vi "iTCread.vi"(0 "VISA resource name":refnum<visa-resource-name>, 1 "iTCreadCtrl":T1, 3 "error in (no error)":errorcluster) -> (7 "VISA resource name out":refnum<visa-resource-name>, 8 "number":dbl, 9 "read buffer":string, 10 "error out":errorcluster)   [LabVIEW 2021]
uses:
  controls/iTCreadCtrl.ctl
  <vilib>/regexp/Match Regular Expression.xnode
panel:
  out "read buffer 2":string
  out "after match":string
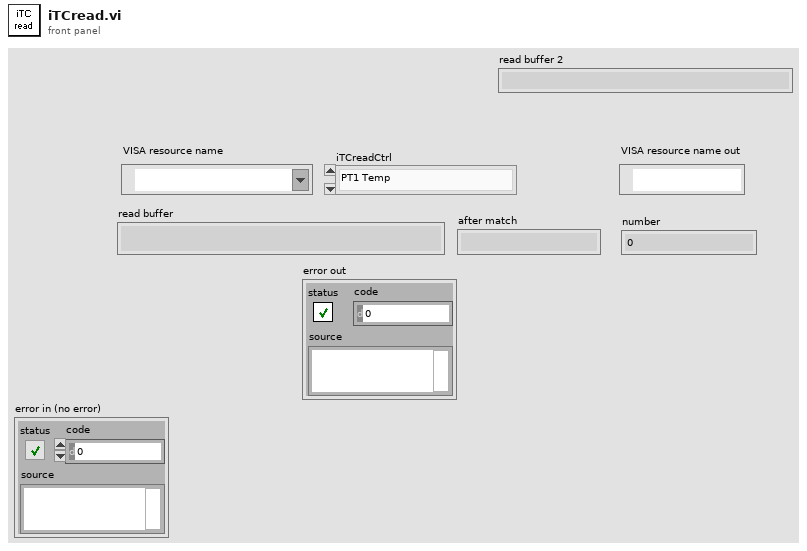
[diagram p1: front panel]
types:
  T1 = typedef "iTCreadCtrl.ctl" = enum16{"PT1 Temp", "PT2 Temp", "Sample Temp", "VTI Temp", "Needle Valve", "VTI Heater Power", "Sample Heater Power", "VTI Pressure"}
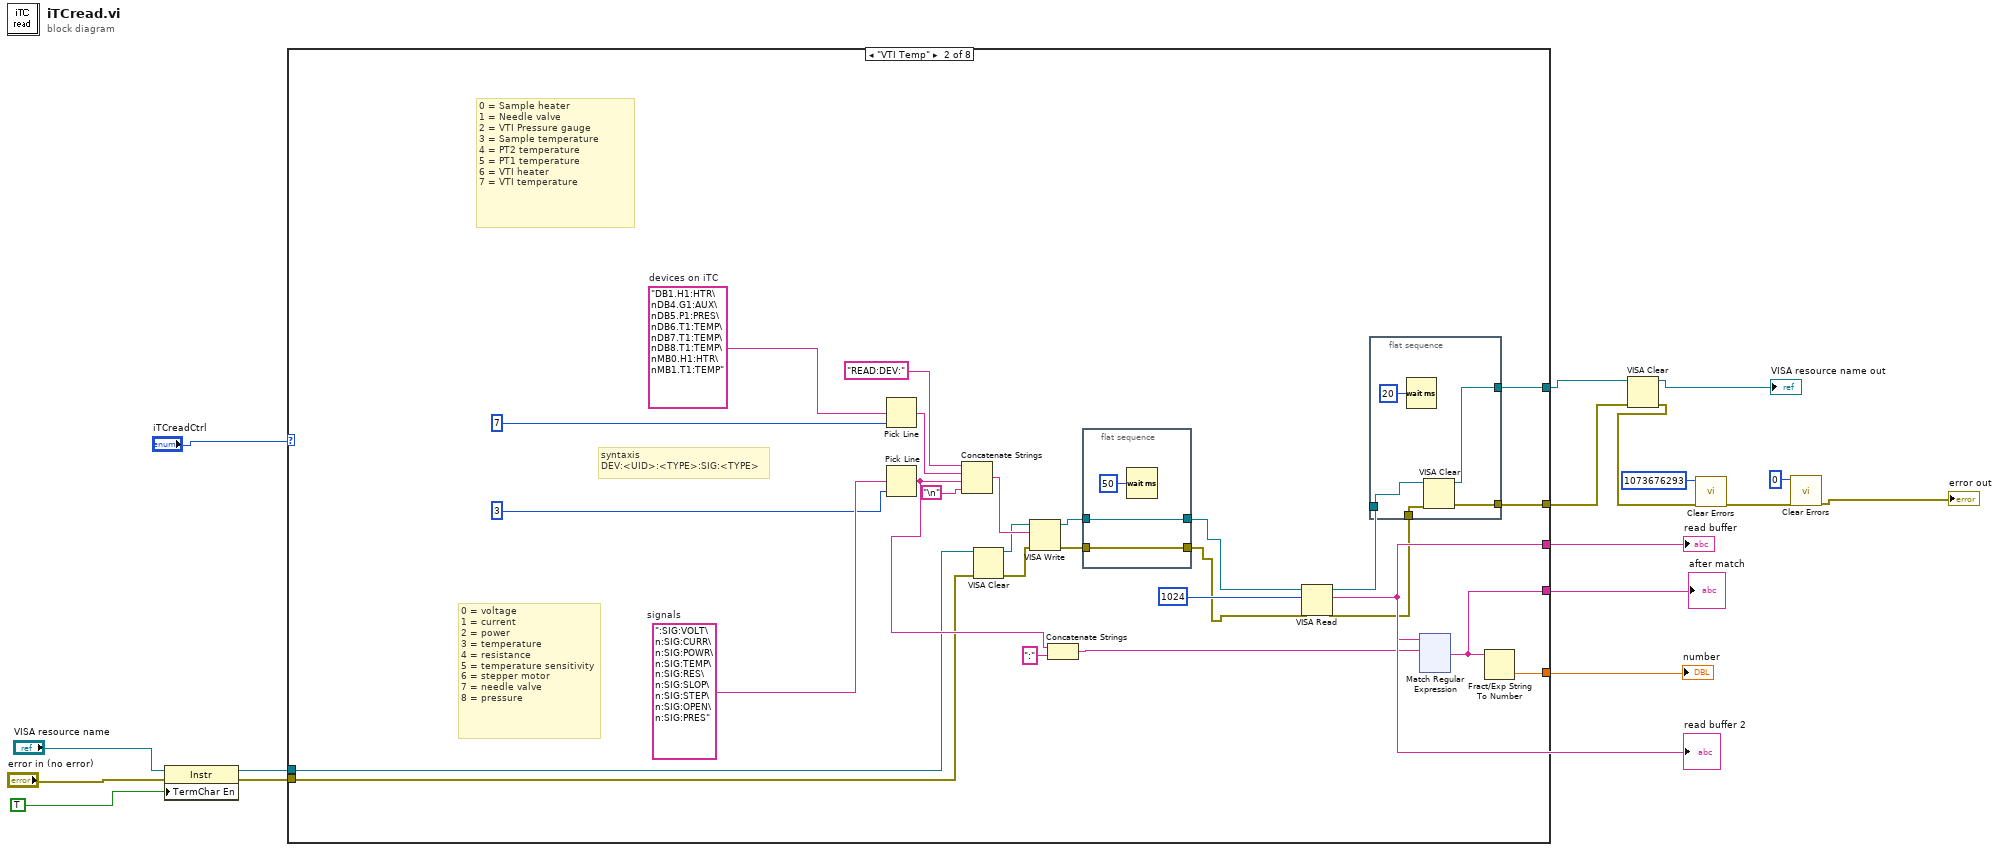
[diagram p0: block diagram]
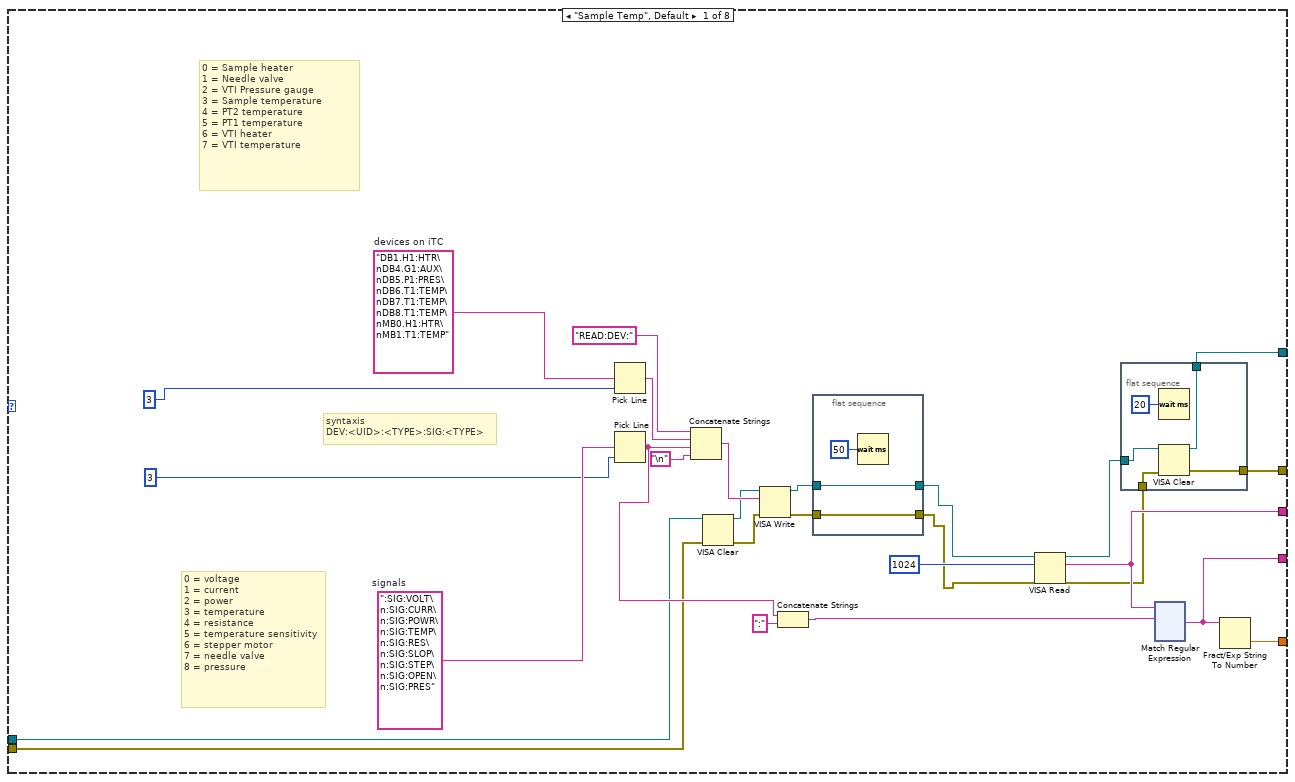
[diagram p2: hidden frame]
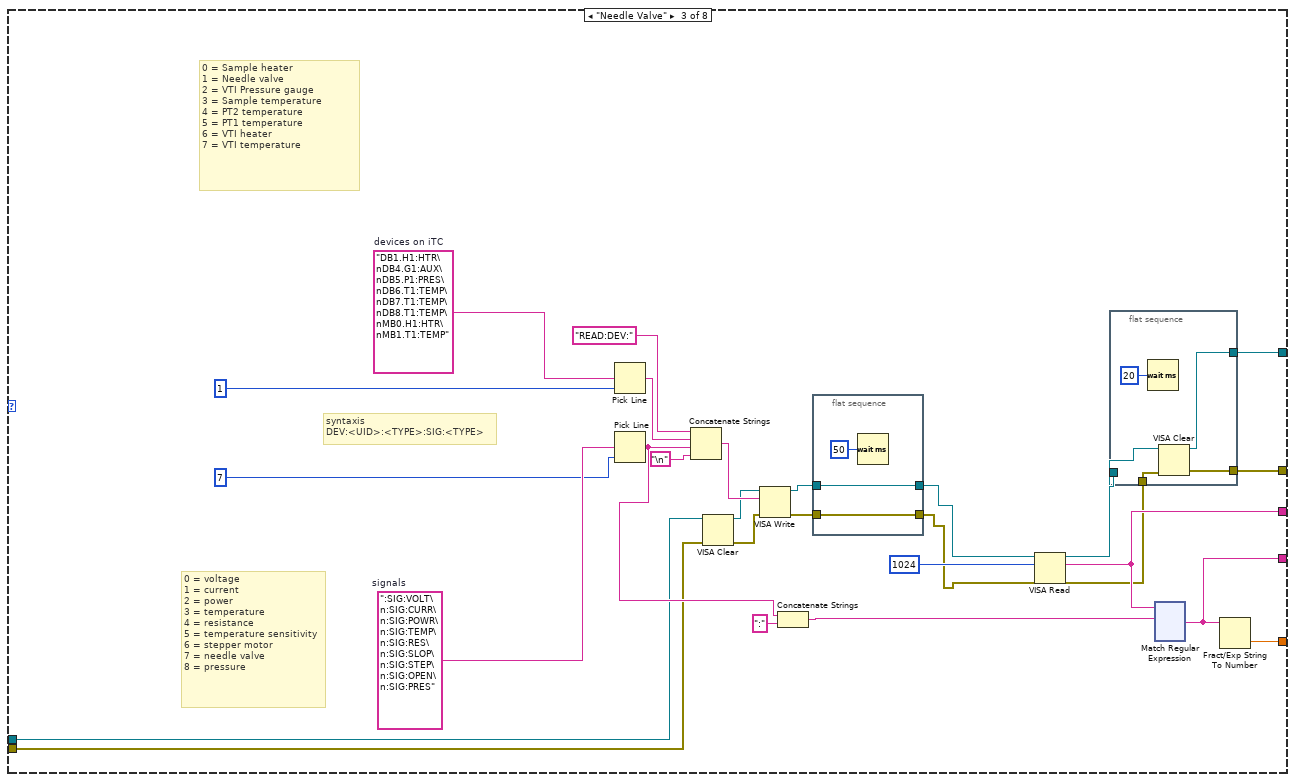
[diagram p3: hidden frame]
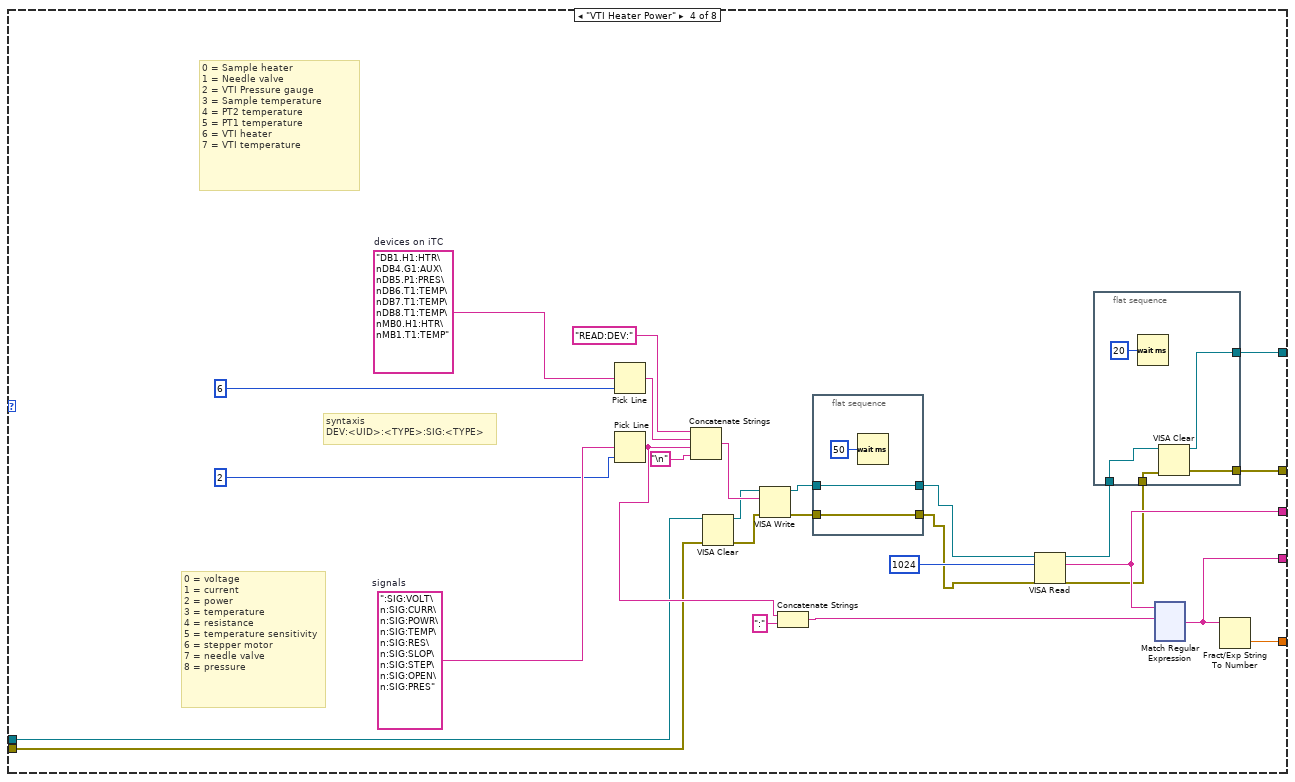
[diagram p4: hidden frame]
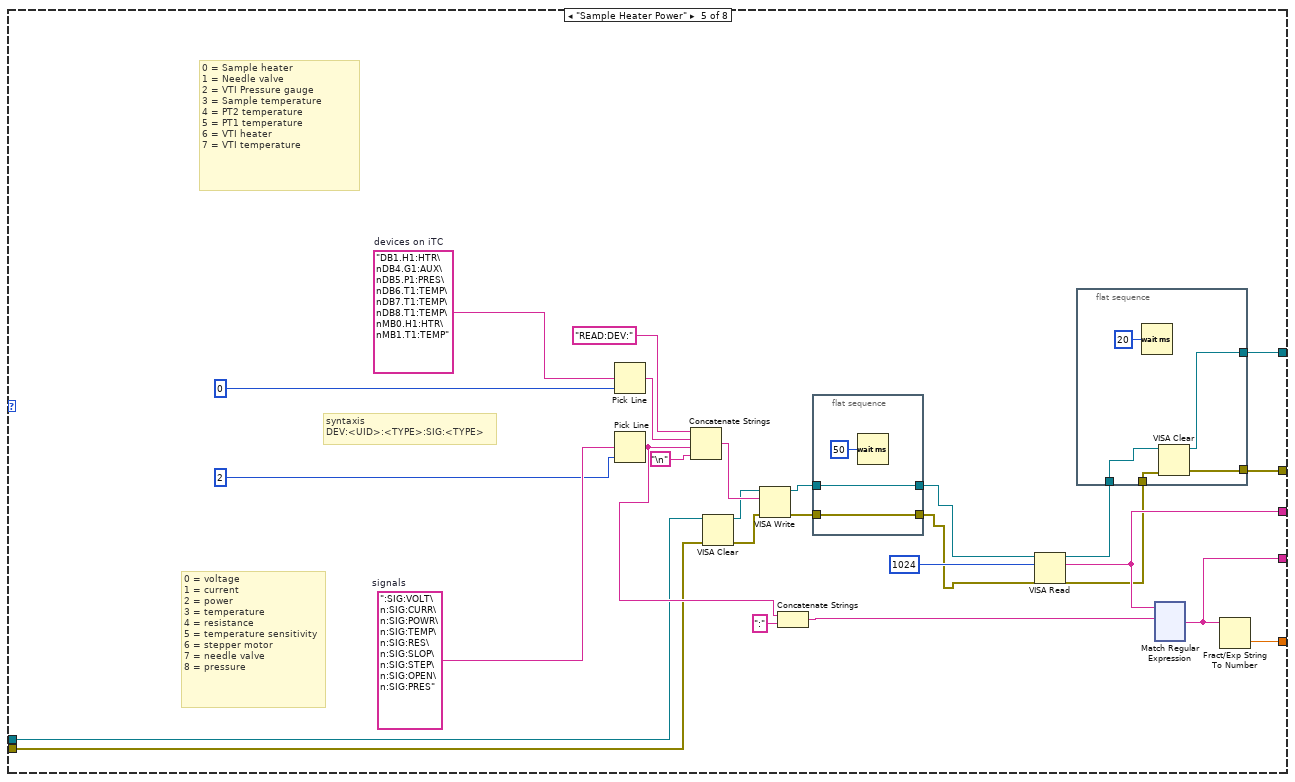
[diagram p5: hidden frame]
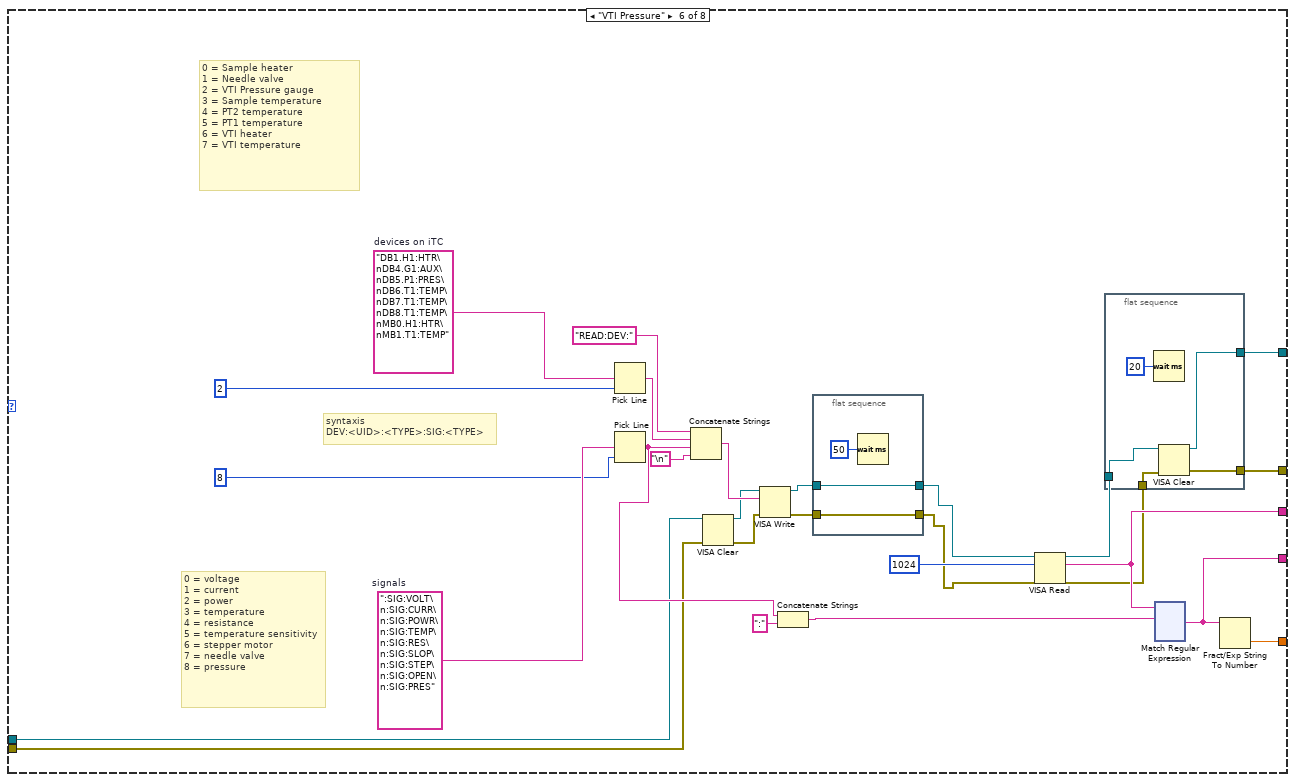
[diagram p6: hidden frame]
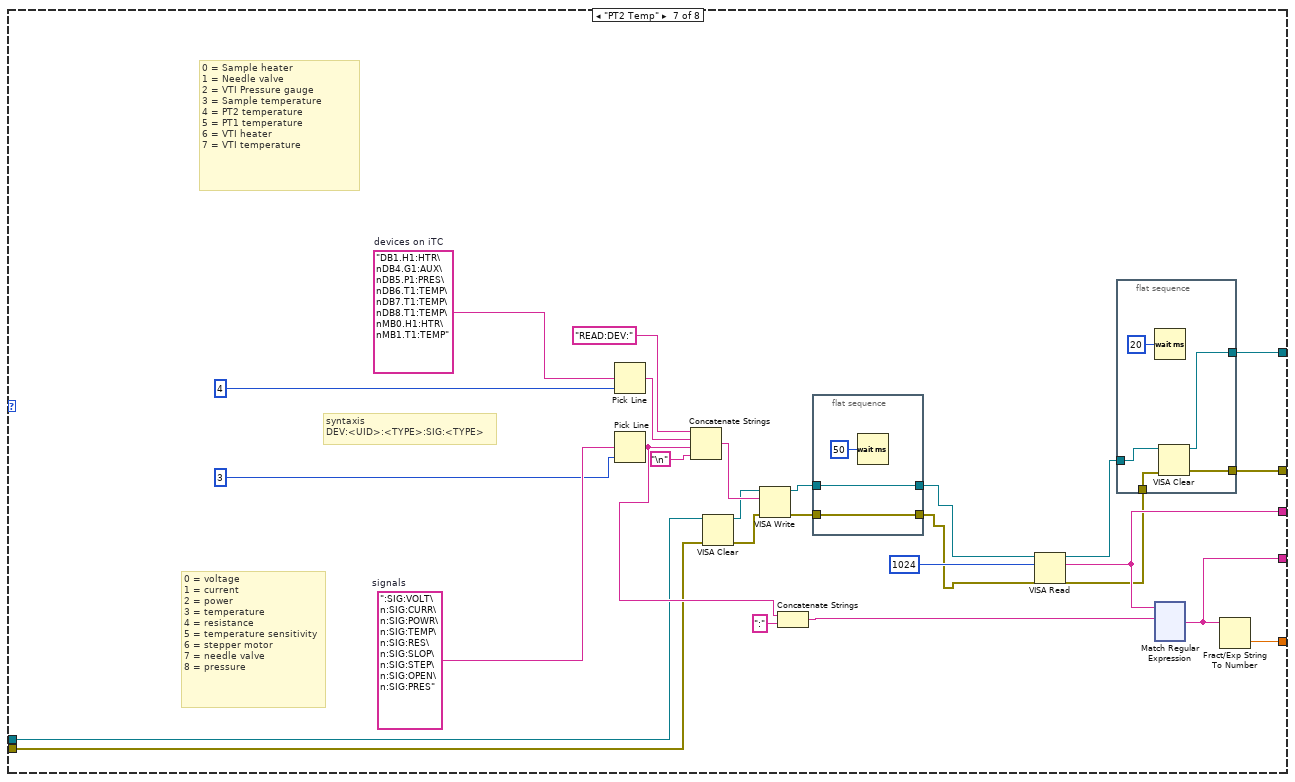
[diagram p7: hidden frame]
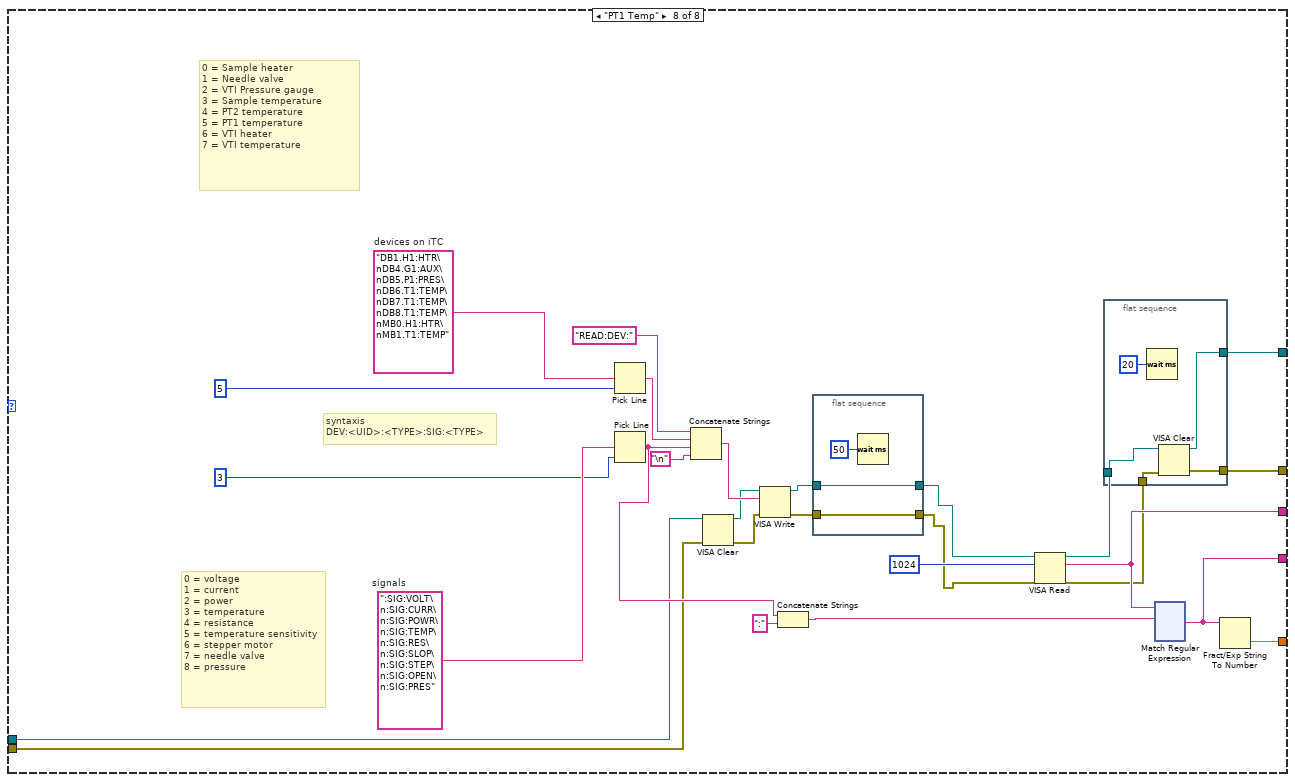
[diagram p8: hidden frame]
diagram:
  n1 = property class="Instr"(reference="VISA resource name", error in="error in (no error)", "TermChar En"=TRUE ("Message Based Settings:Termination Character Enable")) -> (reference out=w11:refnum<visa-resource-name>, error out=w12:errorcluster)
  n2 = case shown="\"VTI Temp\"" "iTCreadCtrl" {
    tunnel: [w44 w196 w348 w500 w652 w804 w956 w1108] -> w17
    tunnel: [w43 w195 w347 w499 w651 w803 w955 w1107] -> w16
    tunnel: [w42 w194 w346 w498 w650 w802 w954 w1106] -> w15
    tunnel: [w41 w193 w345 w497 w649 w801 w953 w1105] -> w2
    tunnel: [w40 w192 w344 w496 w648 w800 w952 w1104] -> w4
    tunnel: w12 -> [w23 w175 w327 w479 w631 w783 w935 w1087]
    tunnel: w11 -> [w22 w174 w326 w478 w630 w782 w934 w1086]
    frame "Sample Temp", Default {
      w36 = ":SIG:VOLT\n:SIG:CURR\n:SIG:POWR\n:SIG:TEMP\n:SIG:RES\n:SIG:SLOP\n:SIG:STEP\n:SIG:OPEN\n:SIG:PRES"  # signals
      w39 = "DB1.H1:HTR\nDB4.G1:AUX\nDB5.P1:PRES\nDB6.T1:TEMP\nDB7.T1:TEMP\nDB8.T1:TEMP\nMB0.H1:HTR\nMB1.T1:TEMP"  # devices on iTC
      # "0 = Sample heater\n1 = Needle valve\n2 = VTI Pressure gauge\n3 = Sample temperature\n4 = PT2 temperature\n5 = PT1 temperature\n6 = VTI heater\n7 = VTI temperature"
      # "0 = voltage\n1 = current\n2 = power\n3 = temperature\n4 = resistance\n5 = temperature sensitivity\n6 = stepper motor\n7 = needle valve\n8 = pressure"
      # "syntaxis\nDEV:<UID>:<TYPE>:SIG:<TYPE>"
      n3 = Pick Line(multi-line string=w39, line index=3) -> (output string=w37:string)  [unwired: 1 in]
      n4 = Pick Line(multi-line string=w36, line index=3) -> (output string=w33:string)  [unwired: 1 in]
      n5 = Concatenate Strings("READ:DEV:" ("write buffer"), w37, w33, "\n") -> (w35:string)
      n6 = VISA Clear(VISA resource name=w22, error in (no error)=w23) -> (VISA resource name out=w26:refnum<visa-resource-name>, error out=w27:errorcluster)
      n7 = VISA Write(VISA resource name=w26, write buffer=w35, error in (no error)=w27) -> (VISA resource name out=w21:refnum<visa-resource-name>, error out=w20:errorcluster)  [unwired: 1 out]
      n8 = Concatenate Strings(w33, ":" ("string")) -> (w32:string)
      n9 = flat-sequence {
        tunnel: w21 -> [w52]
        tunnel: w20 -> [w51]
        tunnel: [w52] -> w19
        tunnel: [w51] -> w18
        frame #0 {
          n10 = Wait (ms)(milliseconds to wait=u32 50) -> ()  [unwired: 1 out]
        }
      }
      n11 = VISA Read(VISA resource name=w19, byte count=u32 1024, error in (no error)=w18) -> (VISA resource name out=w25:refnum<visa-resource-name>, read buffer=w42:string, error out=w28:errorcluster)  [unwired: 1 out]
      n12 = flat-sequence {
        tunnel: [w49] -> w41
        tunnel: [w48] -> w40
        tunnel: w28 -> [w47]
        tunnel: w25 -> [w46]
        frame #0 {
          n13 = Wait (ms)(milliseconds to wait=u32 20) -> ()  [unwired: 1 out]
          n14 = VISA Clear(VISA resource name=w46, error in (no error)=w47) -> (VISA resource name out=w48:refnum<visa-resource-name>, error out=w49:errorcluster)
        }
      }
      n15 = xnode "Match Regular Expression"("input string"=w42, "regular expression"=w32) -> ("after match"=w44:string)  [unwired: 4 in, 4 out]
      n16 = Fract/Exp String To Number(string=w44) -> (number=w43:dbl)  [unwired: 3 in, 1 out]
    }
    frame "VTI Temp" {
      w188 = ":SIG:VOLT\n:SIG:CURR\n:SIG:POWR\n:SIG:TEMP\n:SIG:RES\n:SIG:SLOP\n:SIG:STEP\n:SIG:OPEN\n:SIG:PRES"  # signals
      w191 = "DB1.H1:HTR\nDB4.G1:AUX\nDB5.P1:PRES\nDB6.T1:TEMP\nDB7.T1:TEMP\nDB8.T1:TEMP\nMB0.H1:HTR\nMB1.T1:TEMP"  # devices on iTC
      # "0 = Sample heater\n1 = Needle valve\n2 = VTI Pressure gauge\n3 = Sample temperature\n4 = PT2 temperature\n5 = PT1 temperature\n6 = VTI heater\n7 = VTI temperature"
      # "0 = voltage\n1 = current\n2 = power\n3 = temperature\n4 = resistance\n5 = temperature sensitivity\n6 = stepper motor\n7 = needle valve\n8 = pressure"
      # "syntaxis\nDEV:<UID>:<TYPE>:SIG:<TYPE>"
      n17 = Pick Line(multi-line string=w191, line index=7) -> (output string=w189:string)  [unwired: 1 in]
      n18 = Pick Line(multi-line string=w188, line index=3) -> (output string=w185:string)  [unwired: 1 in]
      n19 = Concatenate Strings("READ:DEV:" ("write buffer"), w189, w185, "\n") -> (w187:string)
      n20 = VISA Clear(VISA resource name=w174, error in (no error)=w175) -> (VISA resource name out=w178:refnum<visa-resource-name>, error out=w179:errorcluster)
      n21 = VISA Write(VISA resource name=w178, write buffer=w187, error in (no error)=w179) -> (VISA resource name out=w173:refnum<visa-resource-name>, error out=w172:errorcluster)  [unwired: 1 out]
      n22 = Concatenate Strings(w185, ":" ("string")) -> (w184:string)
      n23 = flat-sequence {
        tunnel: w173 -> [w204]
        tunnel: w172 -> [w203]
        tunnel: [w204] -> w171
        tunnel: [w203] -> w170
        frame #0 {
          n24 = Wait (ms)(milliseconds to wait=u32 50) -> ()  [unwired: 1 out]
        }
      }
      n25 = VISA Read(VISA resource name=w171, byte count=u32 1024, error in (no error)=w170) -> (VISA resource name out=w177:refnum<visa-resource-name>, read buffer=w194:string, error out=w180:errorcluster)  [unwired: 1 out]
      n26 = flat-sequence {
        tunnel: [w201] -> w193
        tunnel: [w200] -> w192
        tunnel: w180 -> [w199]
        tunnel: w177 -> [w198]
        frame #0 {
          n27 = Wait (ms)(milliseconds to wait=u32 20) -> ()  [unwired: 1 out]
          n28 = VISA Clear(VISA resource name=w198, error in (no error)=w199) -> (VISA resource name out=w200:refnum<visa-resource-name>, error out=w201:errorcluster)
        }
      }
      n29 = xnode "Match Regular Expression"("input string"=w194, "regular expression"=w184) -> ("after match"=w196:string)  [unwired: 4 in, 4 out]
      n30 = Fract/Exp String To Number(string=w196) -> (number=w195:dbl)  [unwired: 3 in, 1 out]
    }
    frame "Needle Valve" {
      w340 = ":SIG:VOLT\n:SIG:CURR\n:SIG:POWR\n:SIG:TEMP\n:SIG:RES\n:SIG:SLOP\n:SIG:STEP\n:SIG:OPEN\n:SIG:PRES"  # signals
      w343 = "DB1.H1:HTR\nDB4.G1:AUX\nDB5.P1:PRES\nDB6.T1:TEMP\nDB7.T1:TEMP\nDB8.T1:TEMP\nMB0.H1:HTR\nMB1.T1:TEMP"  # devices on iTC
      # "0 = Sample heater\n1 = Needle valve\n2 = VTI Pressure gauge\n3 = Sample temperature\n4 = PT2 temperature\n5 = PT1 temperature\n6 = VTI heater\n7 = VTI temperature"
      # "0 = voltage\n1 = current\n2 = power\n3 = temperature\n4 = resistance\n5 = temperature sensitivity\n6 = stepper motor\n7 = needle valve\n8 = pressure"
      # "syntaxis\nDEV:<UID>:<TYPE>:SIG:<TYPE>"
      n31 = Pick Line(multi-line string=w343, line index=1) -> (output string=w341:string)  [unwired: 1 in]
      n32 = Pick Line(multi-line string=w340, line index=7) -> (output string=w337:string)  [unwired: 1 in]
      n33 = Concatenate Strings("READ:DEV:" ("write buffer"), w341, w337, "\n") -> (w339:string)
      n34 = VISA Clear(VISA resource name=w326, error in (no error)=w327) -> (VISA resource name out=w330:refnum<visa-resource-name>, error out=w331:errorcluster)
      n35 = VISA Write(VISA resource name=w330, write buffer=w339, error in (no error)=w331) -> (VISA resource name out=w325:refnum<visa-resource-name>, error out=w324:errorcluster)  [unwired: 1 out]
      n36 = Concatenate Strings(w337, ":" ("string")) -> (w336:string)
      n37 = flat-sequence {
        tunnel: w325 -> [w356]
        tunnel: w324 -> [w355]
        tunnel: [w356] -> w323
        tunnel: [w355] -> w322
        frame #0 {
          n38 = Wait (ms)(milliseconds to wait=u32 50) -> ()  [unwired: 1 out]
        }
      }
      n39 = VISA Read(VISA resource name=w323, byte count=u32 1024, error in (no error)=w322) -> (VISA resource name out=w329:refnum<visa-resource-name>, read buffer=w346:string, error out=w332:errorcluster)  [unwired: 1 out]
      n40 = flat-sequence {
        tunnel: [w353] -> w345
        tunnel: [w352] -> w344
        tunnel: w332 -> [w351]
        tunnel: w329 -> [w350]
        frame #0 {
          n41 = Wait (ms)(milliseconds to wait=u32 20) -> ()  [unwired: 1 out]
          n42 = VISA Clear(VISA resource name=w350, error in (no error)=w351) -> (VISA resource name out=w352:refnum<visa-resource-name>, error out=w353:errorcluster)
        }
      }
      n43 = xnode "Match Regular Expression"("input string"=w346, "regular expression"=w336) -> ("after match"=w348:string)  [unwired: 4 in, 4 out]
      n44 = Fract/Exp String To Number(string=w348) -> (number=w347:dbl)  [unwired: 3 in, 1 out]
    }
    frame "VTI Heater Power" {
      w492 = ":SIG:VOLT\n:SIG:CURR\n:SIG:POWR\n:SIG:TEMP\n:SIG:RES\n:SIG:SLOP\n:SIG:STEP\n:SIG:OPEN\n:SIG:PRES"  # signals
      w495 = "DB1.H1:HTR\nDB4.G1:AUX\nDB5.P1:PRES\nDB6.T1:TEMP\nDB7.T1:TEMP\nDB8.T1:TEMP\nMB0.H1:HTR\nMB1.T1:TEMP"  # devices on iTC
      # "0 = Sample heater\n1 = Needle valve\n2 = VTI Pressure gauge\n3 = Sample temperature\n4 = PT2 temperature\n5 = PT1 temperature\n6 = VTI heater\n7 = VTI temperature"
      # "0 = voltage\n1 = current\n2 = power\n3 = temperature\n4 = resistance\n5 = temperature sensitivity\n6 = stepper motor\n7 = needle valve\n8 = pressure"
      # "syntaxis\nDEV:<UID>:<TYPE>:SIG:<TYPE>"
      n45 = Pick Line(multi-line string=w495, line index=6) -> (output string=w493:string)  [unwired: 1 in]
      n46 = Pick Line(multi-line string=w492, line index=2) -> (output string=w489:string)  [unwired: 1 in]
      n47 = Concatenate Strings("READ:DEV:" ("write buffer"), w493, w489, "\n") -> (w491:string)
      n48 = VISA Clear(VISA resource name=w478, error in (no error)=w479) -> (VISA resource name out=w482:refnum<visa-resource-name>, error out=w483:errorcluster)
      n49 = VISA Write(VISA resource name=w482, write buffer=w491, error in (no error)=w483) -> (VISA resource name out=w477:refnum<visa-resource-name>, error out=w476:errorcluster)  [unwired: 1 out]
      n50 = Concatenate Strings(w489, ":" ("string")) -> (w488:string)
      n51 = flat-sequence {
        tunnel: w477 -> [w508]
        tunnel: w476 -> [w507]
        tunnel: [w508] -> w475
        tunnel: [w507] -> w474
        frame #0 {
          n52 = Wait (ms)(milliseconds to wait=u32 50) -> ()  [unwired: 1 out]
        }
      }
      n53 = VISA Read(VISA resource name=w475, byte count=u32 1024, error in (no error)=w474) -> (VISA resource name out=w481:refnum<visa-resource-name>, read buffer=w498:string, error out=w484:errorcluster)  [unwired: 1 out]
      n54 = flat-sequence {
        tunnel: [w505] -> w497
        tunnel: [w504] -> w496
        tunnel: w484 -> [w503]
        tunnel: w481 -> [w502]
        frame #0 {
          n55 = Wait (ms)(milliseconds to wait=u32 20) -> ()  [unwired: 1 out]
          n56 = VISA Clear(VISA resource name=w502, error in (no error)=w503) -> (VISA resource name out=w504:refnum<visa-resource-name>, error out=w505:errorcluster)
        }
      }
      n57 = xnode "Match Regular Expression"("input string"=w498, "regular expression"=w488) -> ("after match"=w500:string)  [unwired: 4 in, 4 out]
      n58 = Fract/Exp String To Number(string=w500) -> (number=w499:dbl)  [unwired: 3 in, 1 out]
    }
    frame "Sample Heater Power" {
      w644 = ":SIG:VOLT\n:SIG:CURR\n:SIG:POWR\n:SIG:TEMP\n:SIG:RES\n:SIG:SLOP\n:SIG:STEP\n:SIG:OPEN\n:SIG:PRES"  # signals
      w647 = "DB1.H1:HTR\nDB4.G1:AUX\nDB5.P1:PRES\nDB6.T1:TEMP\nDB7.T1:TEMP\nDB8.T1:TEMP\nMB0.H1:HTR\nMB1.T1:TEMP"  # devices on iTC
      # "0 = Sample heater\n1 = Needle valve\n2 = VTI Pressure gauge\n3 = Sample temperature\n4 = PT2 temperature\n5 = PT1 temperature\n6 = VTI heater\n7 = VTI temperature"
      # "0 = voltage\n1 = current\n2 = power\n3 = temperature\n4 = resistance\n5 = temperature sensitivity\n6 = stepper motor\n7 = needle valve\n8 = pressure"
      # "syntaxis\nDEV:<UID>:<TYPE>:SIG:<TYPE>"
      n59 = Pick Line(multi-line string=w647, line index=0) -> (output string=w645:string)  [unwired: 1 in]
      n60 = Pick Line(multi-line string=w644, line index=2) -> (output string=w641:string)  [unwired: 1 in]
      n61 = Concatenate Strings("READ:DEV:" ("write buffer"), w645, w641, "\n") -> (w643:string)
      n62 = VISA Clear(VISA resource name=w630, error in (no error)=w631) -> (VISA resource name out=w634:refnum<visa-resource-name>, error out=w635:errorcluster)
      n63 = VISA Write(VISA resource name=w634, write buffer=w643, error in (no error)=w635) -> (VISA resource name out=w629:refnum<visa-resource-name>, error out=w628:errorcluster)  [unwired: 1 out]
      n64 = Concatenate Strings(w641, ":" ("string")) -> (w640:string)
      n65 = flat-sequence {
        tunnel: w629 -> [w660]
        tunnel: w628 -> [w659]
        tunnel: [w660] -> w627
        tunnel: [w659] -> w626
        frame #0 {
          n66 = Wait (ms)(milliseconds to wait=u32 50) -> ()  [unwired: 1 out]
        }
      }
      n67 = VISA Read(VISA resource name=w627, byte count=u32 1024, error in (no error)=w626) -> (VISA resource name out=w633:refnum<visa-resource-name>, read buffer=w650:string, error out=w636:errorcluster)  [unwired: 1 out]
      n68 = flat-sequence {
        tunnel: [w657] -> w649
        tunnel: [w656] -> w648
        tunnel: w636 -> [w655]
        tunnel: w633 -> [w654]
        frame #0 {
          n69 = Wait (ms)(milliseconds to wait=u32 20) -> ()  [unwired: 1 out]
          n70 = VISA Clear(VISA resource name=w654, error in (no error)=w655) -> (VISA resource name out=w656:refnum<visa-resource-name>, error out=w657:errorcluster)
        }
      }
      n71 = xnode "Match Regular Expression"("input string"=w650, "regular expression"=w640) -> ("after match"=w652:string)  [unwired: 4 in, 4 out]
      n72 = Fract/Exp String To Number(string=w652) -> (number=w651:dbl)  [unwired: 3 in, 1 out]
    }
    frame "VTI Pressure" {
      w796 = ":SIG:VOLT\n:SIG:CURR\n:SIG:POWR\n:SIG:TEMP\n:SIG:RES\n:SIG:SLOP\n:SIG:STEP\n:SIG:OPEN\n:SIG:PRES"  # signals
      w799 = "DB1.H1:HTR\nDB4.G1:AUX\nDB5.P1:PRES\nDB6.T1:TEMP\nDB7.T1:TEMP\nDB8.T1:TEMP\nMB0.H1:HTR\nMB1.T1:TEMP"  # devices on iTC
      # "0 = Sample heater\n1 = Needle valve\n2 = VTI Pressure gauge\n3 = Sample temperature\n4 = PT2 temperature\n5 = PT1 temperature\n6 = VTI heater\n7 = VTI temperature"
      # "0 = voltage\n1 = current\n2 = power\n3 = temperature\n4 = resistance\n5 = temperature sensitivity\n6 = stepper motor\n7 = needle valve\n8 = pressure"
      # "syntaxis\nDEV:<UID>:<TYPE>:SIG:<TYPE>"
      n73 = Pick Line(multi-line string=w799, line index=2) -> (output string=w797:string)  [unwired: 1 in]
      n74 = Pick Line(multi-line string=w796, line index=8) -> (output string=w793:string)  [unwired: 1 in]
      n75 = Concatenate Strings("READ:DEV:" ("write buffer"), w797, w793, "\n") -> (w795:string)
      n76 = VISA Clear(VISA resource name=w782, error in (no error)=w783) -> (VISA resource name out=w786:refnum<visa-resource-name>, error out=w787:errorcluster)
      n77 = VISA Write(VISA resource name=w786, write buffer=w795, error in (no error)=w787) -> (VISA resource name out=w781:refnum<visa-resource-name>, error out=w780:errorcluster)  [unwired: 1 out]
      n78 = Concatenate Strings(w793, ":" ("string")) -> (w792:string)
      n79 = flat-sequence {
        tunnel: w781 -> [w812]
        tunnel: w780 -> [w811]
        tunnel: [w812] -> w779
        tunnel: [w811] -> w778
        frame #0 {
          n80 = Wait (ms)(milliseconds to wait=u32 50) -> ()  [unwired: 1 out]
        }
      }
      n81 = VISA Read(VISA resource name=w779, byte count=u32 1024, error in (no error)=w778) -> (VISA resource name out=w785:refnum<visa-resource-name>, read buffer=w802:string, error out=w788:errorcluster)  [unwired: 1 out]
      n82 = flat-sequence {
        tunnel: [w809] -> w801
        tunnel: [w808] -> w800
        tunnel: w788 -> [w807]
        tunnel: w785 -> [w806]
        frame #0 {
          n83 = Wait (ms)(milliseconds to wait=u32 20) -> ()  [unwired: 1 out]
          n84 = VISA Clear(VISA resource name=w806, error in (no error)=w807) -> (VISA resource name out=w808:refnum<visa-resource-name>, error out=w809:errorcluster)
        }
      }
      n85 = xnode "Match Regular Expression"("input string"=w802, "regular expression"=w792) -> ("after match"=w804:string)  [unwired: 4 in, 4 out]
      n86 = Fract/Exp String To Number(string=w804) -> (number=w803:dbl)  [unwired: 3 in, 1 out]
    }
    frame "PT2 Temp" {
      w948 = ":SIG:VOLT\n:SIG:CURR\n:SIG:POWR\n:SIG:TEMP\n:SIG:RES\n:SIG:SLOP\n:SIG:STEP\n:SIG:OPEN\n:SIG:PRES"  # signals
      w951 = "DB1.H1:HTR\nDB4.G1:AUX\nDB5.P1:PRES\nDB6.T1:TEMP\nDB7.T1:TEMP\nDB8.T1:TEMP\nMB0.H1:HTR\nMB1.T1:TEMP"  # devices on iTC
      # "0 = Sample heater\n1 = Needle valve\n2 = VTI Pressure gauge\n3 = Sample temperature\n4 = PT2 temperature\n5 = PT1 temperature\n6 = VTI heater\n7 = VTI temperature"
      # "0 = voltage\n1 = current\n2 = power\n3 = temperature\n4 = resistance\n5 = temperature sensitivity\n6 = stepper motor\n7 = needle valve\n8 = pressure"
      # "syntaxis\nDEV:<UID>:<TYPE>:SIG:<TYPE>"
      n87 = Pick Line(multi-line string=w951, line index=4) -> (output string=w949:string)  [unwired: 1 in]
      n88 = Pick Line(multi-line string=w948, line index=3) -> (output string=w945:string)  [unwired: 1 in]
      n89 = Concatenate Strings("READ:DEV:" ("write buffer"), w949, w945, "\n") -> (w947:string)
      n90 = VISA Clear(VISA resource name=w934, error in (no error)=w935) -> (VISA resource name out=w938:refnum<visa-resource-name>, error out=w939:errorcluster)
      n91 = VISA Write(VISA resource name=w938, write buffer=w947, error in (no error)=w939) -> (VISA resource name out=w933:refnum<visa-resource-name>, error out=w932:errorcluster)  [unwired: 1 out]
      n92 = Concatenate Strings(w945, ":" ("string")) -> (w944:string)
      n93 = flat-sequence {
        tunnel: w933 -> [w964]
        tunnel: w932 -> [w963]
        tunnel: [w964] -> w931
        tunnel: [w963] -> w930
        frame #0 {
          n94 = Wait (ms)(milliseconds to wait=u32 50) -> ()  [unwired: 1 out]
        }
      }
      n95 = VISA Read(VISA resource name=w931, byte count=u32 1024, error in (no error)=w930) -> (VISA resource name out=w937:refnum<visa-resource-name>, read buffer=w954:string, error out=w940:errorcluster)  [unwired: 1 out]
      n96 = flat-sequence {
        tunnel: [w961] -> w953
        tunnel: [w960] -> w952
        tunnel: w940 -> [w959]
        tunnel: w937 -> [w958]
        frame #0 {
          n97 = Wait (ms)(milliseconds to wait=u32 20) -> ()  [unwired: 1 out]
          n98 = VISA Clear(VISA resource name=w958, error in (no error)=w959) -> (VISA resource name out=w960:refnum<visa-resource-name>, error out=w961:errorcluster)
        }
      }
      n99 = xnode "Match Regular Expression"("input string"=w954, "regular expression"=w944) -> ("after match"=w956:string)  [unwired: 4 in, 4 out]
      n100 = Fract/Exp String To Number(string=w956) -> (number=w955:dbl)  [unwired: 3 in, 1 out]
    }
    frame "PT1 Temp" {
      w1100 = ":SIG:VOLT\n:SIG:CURR\n:SIG:POWR\n:SIG:TEMP\n:SIG:RES\n:SIG:SLOP\n:SIG:STEP\n:SIG:OPEN\n:SIG:PRES"  # signals
      w1103 = "DB1.H1:HTR\nDB4.G1:AUX\nDB5.P1:PRES\nDB6.T1:TEMP\nDB7.T1:TEMP\nDB8.T1:TEMP\nMB0.H1:HTR\nMB1.T1:TEMP"  # devices on iTC
      # "0 = Sample heater\n1 = Needle valve\n2 = VTI Pressure gauge\n3 = Sample temperature\n4 = PT2 temperature\n5 = PT1 temperature\n6 = VTI heater\n7 = VTI temperature"
      # "0 = voltage\n1 = current\n2 = power\n3 = temperature\n4 = resistance\n5 = temperature sensitivity\n6 = stepper motor\n7 = needle valve\n8 = pressure"
      # "syntaxis\nDEV:<UID>:<TYPE>:SIG:<TYPE>"
      n101 = Pick Line(multi-line string=w1103, line index=5) -> (output string=w1101:string)  [unwired: 1 in]
      n102 = Pick Line(multi-line string=w1100, line index=3) -> (output string=w1097:string)  [unwired: 1 in]
      n103 = Concatenate Strings("READ:DEV:" ("write buffer"), w1101, w1097, "\n") -> (w1099:string)
      n104 = VISA Clear(VISA resource name=w1086, error in (no error)=w1087) -> (VISA resource name out=w1090:refnum<visa-resource-name>, error out=w1091:errorcluster)
      n105 = VISA Write(VISA resource name=w1090, write buffer=w1099, error in (no error)=w1091) -> (VISA resource name out=w1085:refnum<visa-resource-name>, error out=w1084:errorcluster)  [unwired: 1 out]
      n106 = Concatenate Strings(w1097, ":" ("string")) -> (w1096:string)
      n107 = flat-sequence {
        tunnel: w1085 -> [w1116]
        tunnel: w1084 -> [w1115]
        tunnel: [w1116] -> w1083
        tunnel: [w1115] -> w1082
        frame #0 {
          n108 = Wait (ms)(milliseconds to wait=u32 50) -> ()  [unwired: 1 out]
        }
      }
      n109 = VISA Read(VISA resource name=w1083, byte count=u32 1024, error in (no error)=w1082) -> (VISA resource name out=w1089:refnum<visa-resource-name>, read buffer=w1106:string, error out=w1092:errorcluster)  [unwired: 1 out]
      n110 = flat-sequence {
        tunnel: [w1113] -> w1105
        tunnel: [w1112] -> w1104
        tunnel: w1092 -> [w1111]
        tunnel: w1089 -> [w1110]
        frame #0 {
          n111 = Wait (ms)(milliseconds to wait=u32 20) -> ()  [unwired: 1 out]
          n112 = VISA Clear(VISA resource name=w1110, error in (no error)=w1111) -> (VISA resource name out=w1112:refnum<visa-resource-name>, error out=w1113:errorcluster)
        }
      }
      n113 = xnode "Match Regular Expression"("input string"=w1106, "regular expression"=w1096) -> ("after match"=w1108:string)  [unwired: 4 in, 4 out]
      n114 = Fract/Exp String To Number(string=w1108) -> (number=w1107:dbl)  [unwired: 3 in, 1 out]
    }
  }
  "read buffer" <- w15
  "after match" <- w17
  "number" <- w16
  "read buffer 2" <- w15
  n115 = VISA Clear(VISA resource name=w4, error in (no error)=w2) -> (VISA resource name out=→"VISA resource name out":refnum<visa-resource-name>, error out=w1:errorcluster)
  n116 = call <vilib>:"Clear Errors.vi"("error in (no error)"=w1, "specific error code to clear (0: all)"=1073676293) -> ("error out"=w7:errorcluster)  [unwired: 4 in, 1 out]
  n117 = call <vilib>:"Clear Errors.vi"("error in (no error)"=w7, "specific error code to clear (0: all)"=0) -> ("error out"=→"error out":errorcluster)  [unwired: 4 in, 1 out]
